vi "T14.vi"(2 "Parametry Ziemi":T1={"a - półoś duża"=6378137.0, "b - półoś mała"=6356752.3141999999998} {"b - półoś mała" format="%_20f"; "a - półoś duża" format="%_20g"}, 3 "fi'":ext) -> (7 "T14":ext)   [LabVIEW 2012, in "Biblioteka moduł map v3.lvlib" / "Konwersja wsp.lvlib" / "UTM.lvlib" / "Konwersja z UTM na wsp geograficzne.lvlib"]
uses:
  Konwersja z UTM na wsp geograficzne.lvlib
  UTM.lvlib
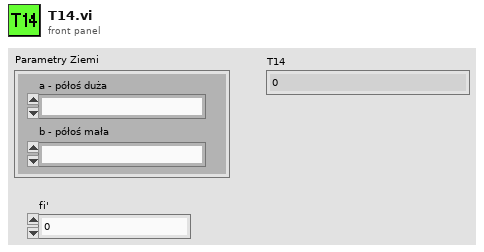
[diagram p1: front panel]
types:
  T1 = cluster{"a - półoś duża":ext, "b - półoś mała":ext}
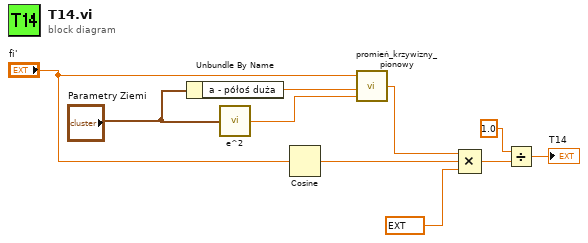
[diagram p0: block diagram]
diagram:
  n1 = Unbundle By Name("Parametry Ziemi") -> ("a - półoś duża"=w1:ext)
  n2 = call "e^2.vi"("Parametry Ziemi"="Parametry Ziemi") -> ("e^2"=w3:ext)  [unwired: 4 in]
  n3 = Cosine(x="fi'") -> (cos(x)=w4:ext)
  n4 = call "promień_krzywizny_pionowy.vi"("e^2"=w3, "a"=w1, "fi[rad]"="fi'") -> ("Promien krzywizny równoleżnika"=w9:ext)  [unwired: 2 in]
  n5 = Compound Arithmetic op=MULTIPLY(w9, w4, ext 0.9996 ("k0")) -> (w7:ext)
  n6 = Divide(x=1.0, y=w7) -> (x/y=→"T14":ext)
